vi "Main.vi"() -> ()   [LabVIEW 2026]
uses:
  <instrlib>/Agilent 34970/Agilent 34970.lvlib
  <vilib>/Utility/TDMS File Viewer/NI_TDMS File Viewer.lvlib
panel:
  in  "Allow cellbalansing":bool
  out "error out":errorcluster
  out "Over under curent":bool
  out "Overehat":bool
  out "Temp":dbl[](array[slide]) scale=0.0..100.0
  out "Current":dbl(knob) scale=-200.0..200.0
  in  "Switching":refnum<visa-resource-name>="GPIB0::9::INSTR"
  out "Total Voltage":dbl(knob) scale=3.0..34.0
  in  "Voltage":refnum<visa-resource-name>="GPIB0::9::INSTR"
  in  "stop":bool
  out "Cell Values":T1(array[cluster])
  # "Befor runninng Selet your switching addresses"
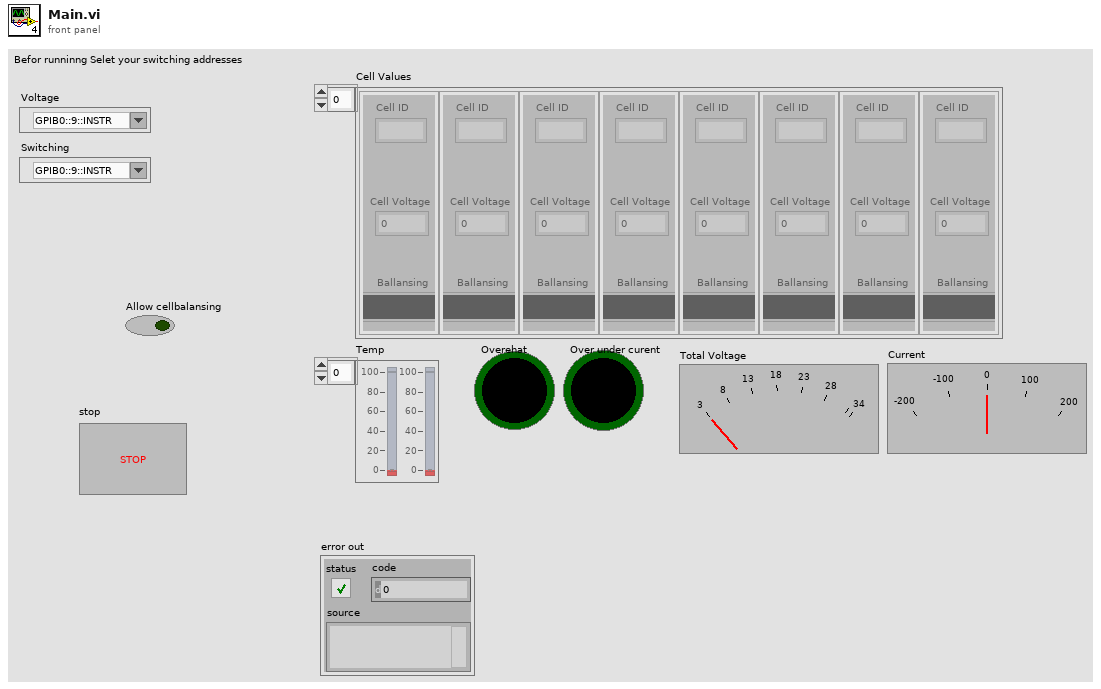
[diagram p1: front panel]
types:
  T1 = cluster{"Ballansing":bool, "Cell Voltage":dbl, "Cell ID":string}[]
  T2 = enum16{"open", "open or create", "create or replace", "create", "open (read-only)"}
  T3 = cluster{"Timeout Value (10000)":u32, "Baud Rate (57600)":enum16{"1200", "2400", "4800", "9600", "19200", "38400", "57600", "115200"}, "Flow Control (1:XON/XOFF)":enum16{"None", "XON / XOFF", "RTS / CTS", "DTR / DSR"}}
  T4 = cluster{"Cell Values":cluster{"Ballansing":bool, "Cell Voltage":dbl, "Cell Id":string}[], "Temp":dbl[], "Curent":dbl, "Overehat":bool, "Over under curent":bool, "Time":timestamp}
  T5 = cluster{"Voltage":dbl[], "Temp":dbl[], "Curent":dbl, "Time":timestamp}
  T6 = cluster{"Ballansing":bool, "Cell Voltage":dbl, "Cell Id":string}[]
  T7 = cluster{"Ballansing":bool, "Cell Voltage":dbl, "Cell Id":string}
  T8 = enum16{"100 mV", "1 V", "10 V", "100 V", "300 V", "Auto", "Minimum", "Maximum"}
  T9 = enum16{"4 1/2", "5 1/2", "6 1/2", "Least", "Highest", "Default"}
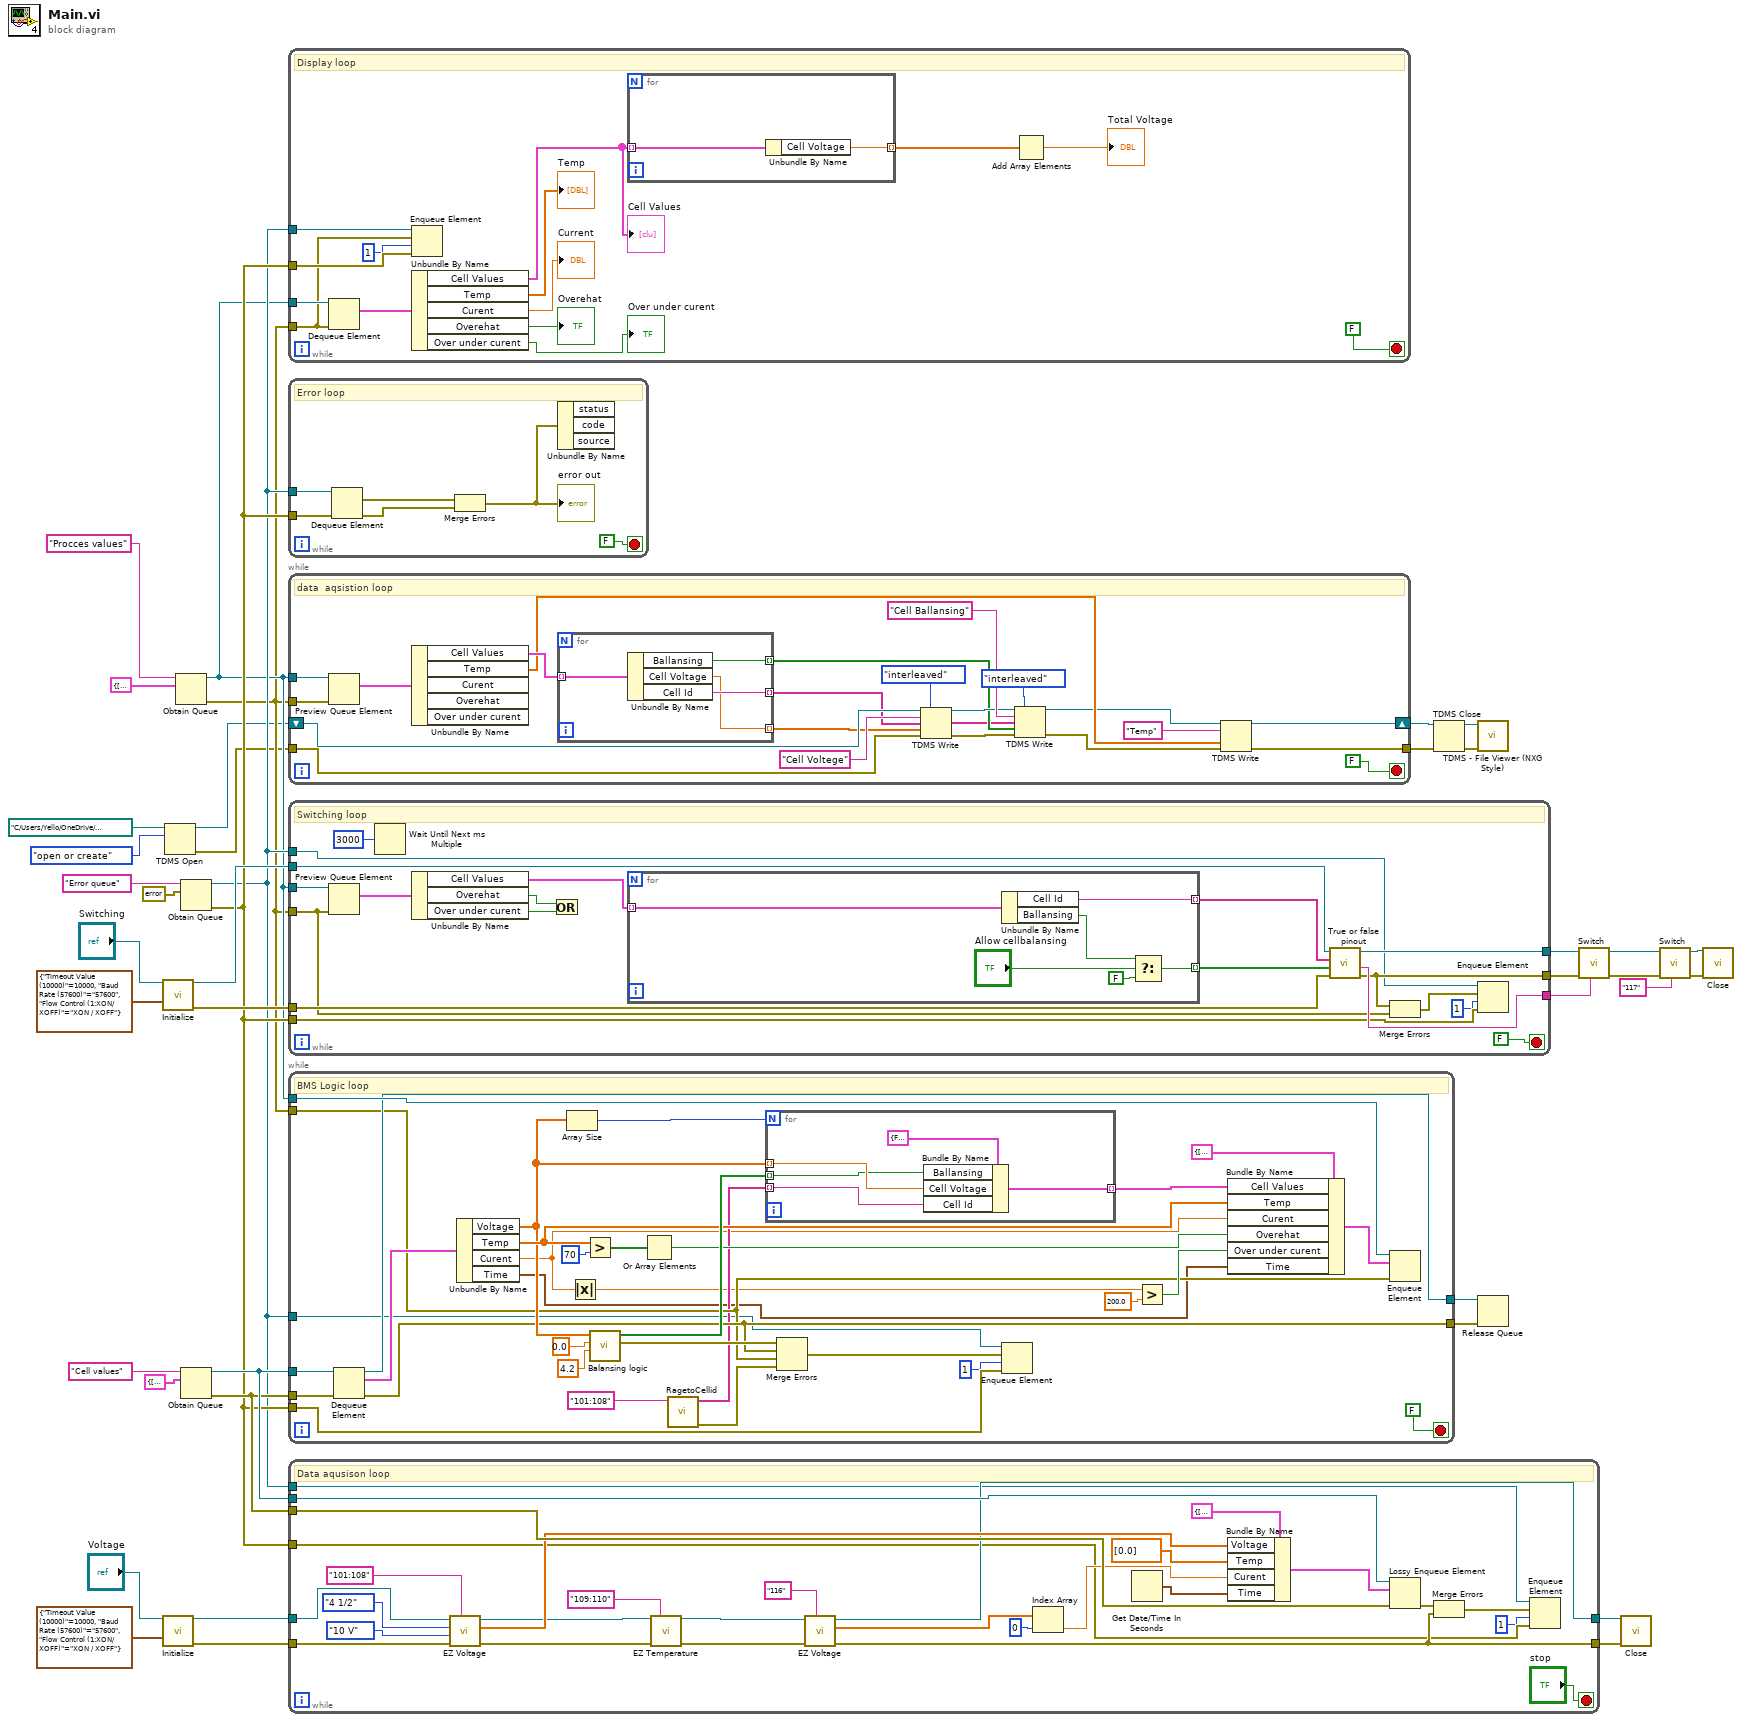
[diagram p0: block diagram]
diagram:
  n1 = call <instrlib>:"Initialize.vi"("VISA Resource Name"="Switching", "Serial Port Configuration"=T3 {"Timeout Value (10000)"=10000, "Baud Rate (57600)"=enum."57600", "Flow Control (1:XON/XOFF)"=enum."XON / XOFF"}) -> ("VISA Resource Name Out"=w24:refnum<visa-resource-name>, "error out"=w23:errorcluster)  [unwired: 12 in]
  n2 = call <instrlib>:"Initialize.vi"("VISA Resource Name"="Voltage", "Serial Port Configuration"=T3 {"Timeout Value (10000)"=10000, "Baud Rate (57600)"=enum."57600", "Flow Control (1:XON/XOFF)"=enum."XON / XOFF"}) -> ("VISA Resource Name Out"=w36:refnum<visa-resource-name>, "error out"=w35:errorcluster)  [unwired: 12 in]
  n3 = TDMS Open(10:T2."open or create" ("operation (0:open)"), 11:path "C:/Users/Yello/OneDrive/Dokumenter/MVBL-BMS/.MVBL-bms.UserState/Log/data" ("file path")) -> (0:w6:errorcluster, 3:w7:refnum<k34>)  [unwired: 5 in]
  n4 = Obtain Queue(name (unnamed)="Procces values", element data type=T4 {"Cell Values"=[{"Ballansing"=FALSE, "Cell Voltage"=0.0, "Cell Id"=""}], "Temp"=[], "Curent"=0.0, "Overehat"=FALSE, "Over under curent"=FALSE, "Time"=timestamp(0 s since 1904-01-01)}) -> (queue out=w10:refnum<queue>, error out=w9:errorcluster)  [unwired: 3 in, 1 out]
  n5 = Obtain Queue(name (unnamed)="Error queue", element data type=errorcluster {"status"=FALSE, "code"=0, "source"=""} ("error constant")) -> (queue out=w11:refnum<queue>, error out=w12:errorcluster)  [unwired: 3 in, 1 out]
  n6 = Obtain Queue(name (unnamed)="Cell values", element data type=T5 {"Voltage"=[], "Temp"=[], "Curent"=0.0, "Time"=timestamp(0 s since 1904-01-01)}) -> (queue out=w38:refnum<queue>, error out=w37:errorcluster)  [unwired: 3 in, 1 out]
  n7 = while {
    tunnel: w10 -> [w42]
    tunnel: w9 -> [w41]
    tunnel: w11 -> [w46]
    tunnel: w12 -> [w45]
    stop <- FALSE stop-if-true
    # "Display loop"
    n8 = Dequeue Element(queue=w42, error in (no error)=w41) -> (element=w43:T4)  [unwired: 1 in, 3 out]
    n9 = Enqueue Element(queue=w46, element=w41, timeout in ms (-1)=1, error in (no error)=w45) -> ()  [unwired: 3 out]
    n10 = Unbundle By Name(w43) -> ("Cell Values"=w54:T6, "Temp"=→"Temp":dbl[], "Curent"=→"Current":dbl, "Overehat"=→"Overehat":bool, "Over under curent"=→"Over under curent":bool)
    "Cell Values" <- w54
    n11 = for {
      tunnel: w54 -> [w56] mode=indexing
      tunnel: [w55] -> w53 mode=indexing
      n12 = Unbundle By Name(w56) -> ("Cell Voltage"=w55:dbl)
    }
    n13 = Add Array Elements(numeric array=w53) -> (sum=→"Total Voltage":dbl)
  }
  n14 = while {
    tunnel: w11 -> [w62]
    tunnel: w12 -> [w61]
    stop <- FALSE stop-if-true
    # "Error loop"
    n15 = Dequeue Element(queue=w62, error in (no error)=w61) -> (element=w60:errorcluster, error out=w59:errorcluster)  [unwired: 1 in, 2 out]
    n16 = Merge Errors(w60, w59) -> (w58:errorcluster)
    "error out" <- w58
    n17 = Unbundle By Name(w58) -> ()  [unwired: 3 out]
  }
  n18 = while {
    tunnel: w10 -> [w83]
    tunnel: w9 -> [w82]
    shift-right: [w67] -> w5
    shift-left: w7 -> [w85]
    tunnel: w6 -> [w84]
    tunnel: [w66] -> w4
    stop <- FALSE stop-if-true
    # "data  aqsistion loop"
    n19 = Preview Queue Element(queue=w83, error in (no error)=w82) -> (element=w80:T4)  [unwired: 1 in, 3 out]
    n20 = Unbundle By Name(w80) -> ("Cell Values"=w79:T6, "Temp"=w70:dbl[])  [unwired: 3 out]
    n21 = for {
      tunnel: w79 -> [w89] mode=indexing
      tunnel: [w88] -> w72 mode=indexing
      tunnel: [w87] -> w73 mode=indexing
      tunnel: [w86] -> w71 mode=indexing
      n22 = Unbundle By Name(w89) -> ("Ballansing"=w86:bool, "Cell Voltage"=w87:dbl, "Cell Id"=w88:string)
    }
    n23 = TDMS Write(0:w85, 1:enum16{"decimated", "interleaved"}."interleaved" ("data layout (0:decimated)"), 5:"Cell Voltege" ("group name in (Untitled)"), 7:w72, 9:w73, 11:w84) -> (4:w77:refnum<k34>, 8:w64:string[], 15:w76:errorcluster)  [unwired: 1 out]
    n24 = TDMS Write(0:w77, 1:enum16{"decimated", "interleaved"}."interleaved" ("data layout (0:decimated)"), 5:"Cell Ballansing" ("group name in (Untitled)"), 7:w64, 9:w71, 11:w76) -> (4:w68:refnum<k34>, 15:w69:errorcluster)  [unwired: 2 out]
    n25 = TDMS Write(0:w68, 5:"Temp" ("group name in (Untitled)"), 9:w70, 11:w69) -> (4:w67:refnum<k34>, 15:w66:errorcluster)  [unwired: 2 in, 2 out]
  }
  n26 = while {
    tunnel: w24 -> [w107]
    tunnel: w23 -> [w108]
    tunnel: [w98] -> w19
    tunnel: [w106] -> w18
    tunnel: w10 -> [w92]
    tunnel: w9 -> [w91]
    tunnel: [w100] -> w20
    tunnel: w11 -> [w97]
    tunnel: w12 -> [w96]
    stop <- FALSE stop-if-true
    # "Switching loop"
    n27 = Preview Queue Element(queue=w92, error in (no error)=w91) -> (element=w93:T4)  [unwired: 1 in, 3 out]
    n28 = Wait Until Next ms Multiple(millisecond multiple=u32 3000) -> ()  [unwired: 1 out]
    n29 = Unbundle By Name(w93) -> ("Cell Values"=w105:T6, "Overehat"=w102:bool, "Over under curent"=w101:bool)
    n30 = Or(x=w102, y=w101) -> ()  [unwired: 1 out]
    n31 = for {
      tunnel: w105 -> [w114] mode=indexing
      tunnel: [w113] -> w104 mode=indexing
      tunnel: [w112] -> w103 mode=indexing
      n32 = Unbundle By Name(w114) -> ("Cell Id"=w113:string, "Ballansing"=w111:bool)
      n33 = Select(t=w111, s="Allow cellbalansing", f=FALSE) -> (s? t:f=w112:bool)
    }
    n34 = call "True or false pinout.vi"("VISA Resource Name"=w107, "Input str"=w104, "State"=w103, "error in (no error)"=w108) -> ("VISA Resource Name Out"=w106:refnum<visa-resource-name>, "Exir str"=w100:string, "error out"=w98:errorcluster)  [unwired: 3 in]
    n35 = Merge Errors(w98, w91) -> (w99:errorcluster)
    n36 = Enqueue Element(queue=w97, element=w99, timeout in ms (-1)=1, error in (no error)=w96) -> ()  [unwired: 3 out]
  }
  n37 = while {
    tunnel: w38 -> [w147]
    tunnel: w37 -> [w146]
    tunnel: w9 -> [w125]
    tunnel: w10 -> [w144]
    tunnel: [w126] -> w27
    tunnel: [w128] -> w28
    tunnel: w11 -> [w118]
    tunnel: w12 -> [w117]
    stop <- FALSE stop-if-true
    # "BMS Logic loop"
    n38 = Dequeue Element(queue=w147, error in (no error)=w146) -> (queue out=w128:refnum<queue>, element=w145:T5, error out=w126:errorcluster)  [unwired: 1 in, 1 out]
    n39 = Unbundle By Name(w145) -> ("Voltage"=w130:dbl[], "Temp"=w135:dbl[], "Curent"=w120:dbl, "Time"=w115:timestamp)
    n40 = Array Size(array=w130) -> (size(s)=w129:i32)
    n41 = Absolute Value(x=w120) -> (abs(x)=w121:dbl)
    n42 = Greater?(x=w135, y=70) -> (0:w134:bool[])
    n43 = call "Balansing logic.vi"("Vmax"=4.2, "Vmin"=0.0, "Voltage"=w130) -> ("error constant"=w127:errorcluster, "Array"=w140:bool[])  [unwired: 7 in]
    n44 = Or Array Elements(Boolean array=w134) -> (logical OR=w133:bool)
    n45 = call "RagetoCellid.vi"("Voltage ID Range"="101:108") -> ("Error out"=w123:errorcluster, "Cell ids"=w124:string[])  [unwired: 9 in]
    n46 = for {
      N: w129 -> [_]
      tunnel: [w152] -> w141 mode=indexing
      tunnel: w130 -> [w150] mode=indexing
      tunnel: w140 -> [w149] mode=indexing
      tunnel: w124 -> [w148] mode=indexing
      n47 = Bundle By Name(cluster=T7 {"Ballansing"=FALSE, "Cell Voltage"=0.0, "Cell Id"=""} ("Cluster"), "Ballansing"=w149, "Cell Voltage"=w150, "Cell Id"=w148) -> (w152:T7)
    }
    n48 = Merge Errors(w127, w126, w125, w123) -> (w119:errorcluster)
    n49 = Enqueue Element(queue=w118, element=w119, timeout in ms (-1)=1, error in (no error)=w117) -> ()  [unwired: 3 out]
    n50 = Greater?(x=w121, y=200.0) -> (0:w137:bool)
    n51 = Bundle By Name(cluster=T4 {"Cell Values"=[{"Ballansing"=FALSE, "Cell Voltage"=0.0, "Cell Id"=""}], "Temp"=[], "Curent"=0.0, "Overehat"=FALSE, "Over under curent"=FALSE, "Time"=timestamp(0 s since 1904-01-01)}, "Cell Values"=w141, "Temp"=w135, "Curent"=w120, "Overehat"=w133, "Over under curent"=w137, "Time"=w115) -> (w143:T4)
    n52 = Enqueue Element(queue=w144, element=w143, error in (no error)=w125) -> ()  [unwired: 1 in, 3 out]
  }
  n53 = while {
    tunnel: w38 -> [w180]
    tunnel: w37 -> [w179]
    tunnel: w36 -> [w175]
    tunnel: w35 -> [w174]
    tunnel: [w164] -> w34
    tunnel: [w161] -> w33
    tunnel: w12 -> [w159]
    tunnel: w11 -> [w158]
    stop <- "stop" stop-if-true
    # "Data aqusison loop"
    n54 = call <instrlib>:"EZ Voltage.vi"("Scan List (empty)"="101:108", "error in (no error)"=w174, "Range (5:Auto)"=T8."10 V", "Resolution (5:Default)"=T9."4 1/2", "VISA Resource Name"=w175) -> ("error out"=w171:errorcluster, "Output Array"=w173:dbl[], "VISA Resource Name Out"=w172:refnum<visa-resource-name>)  [unwired: 4 in]
    n55 = call <instrlib>:"EZ Temperature.vi"("VISA Resource Name"=w172, "Scan List (empty)"="109:110", "error in (no error)"=w171) -> ("VISA Resource Name Out"=w169:refnum<visa-resource-name>, "error out"=w168:errorcluster)  [unwired: 10 in, 1 out]
    n56 = call <instrlib>:"EZ Voltage.vi"("Scan List (empty)"="116", "error in (no error)"=w168, "VISA Resource Name"=w169) -> ("error out"=w161:errorcluster, "Output Array"=w166:dbl[], "VISA Resource Name Out"=w164:refnum<visa-resource-name>)  [unwired: 6 in]
    n57 = Index Array(array=w166, index=0) -> (element=w165:dbl)
    n58 = Get Date/Time In Seconds() -> (seconds since 1Jan1904=w153:timestamp)
    n59 = Bundle By Name(cluster=T5 {"Voltage"=[], "Temp"=[], "Curent"=0.0, "Time"=timestamp(0 s since 1904-01-01)}, "Voltage"=w173, "Temp"=dbl[] [0.0], "Curent"=w165, "Time"=w153) -> (w177:T5)
    n60 = Lossy Enqueue Element(queue=w180, element=w177, error in (no error)=w179) -> (error out=w162:errorcluster)  [unwired: 3 out]
    n61 = Merge Errors(w162, w161) -> (w160:errorcluster)
    n62 = Enqueue Element(queue=w158, element=w160, timeout in ms (-1)=1, error in (no error)=w159) -> ()  [unwired: 3 out]
  }
  n63 = TDMS Close(8:w4, 11:w5) -> (0:w2:errorcluster, 3:w3:path)
  n64 = call <vilib>:"TDMS - File Viewer (NXG Style).vi"("error in"=w2, "file in"=w3) -> ()  [unwired: 8 in, 2 out]
  n65 = Release Queue(queue=w28, error in (no error)=w27) -> ()  [unwired: 1 in, 3 out]
  n66 = call <instrlib>:"Switch.vi"("Channel List(empty)"=w20, "error in (no error)"=w19, "VISA Resource Name"=w18) -> ("error out"=w17:errorcluster, "VISA Resource Name Out"=w14:refnum<visa-resource-name>)  [unwired: 6 in, 1 out]
  n67 = call <instrlib>:"Close.vi"("VISA Resource Name"=w34, "error in (no error)"=w33) -> ()  [unwired: 13 in, 1 out]
  n68 = call <instrlib>:"Switch.vi"("Channel List(empty)"="117", "error in (no error)"=w17, "VISA Resource Name"=w14) -> ("error out"=w16:errorcluster, "VISA Resource Name Out"=w15:refnum<visa-resource-name>)  [unwired: 6 in, 1 out]
  n69 = call <instrlib>:"Close.vi"("VISA Resource Name"=w15, "error in (no error)"=w16) -> ()  [unwired: 13 in, 1 out]
